vi "ABB locked rotor results.vi"(0 "Rated Current":dbl, 9 "Locked rotor test results":dbl[][](array[numeric])) -> (2 "PFr":dbl, 3 "I AVr":dbl, 4 "IUr":dbl, 6 "IVr":dbl, 8 "PWr":dbl, 10 "IWr":dbl, 13 "V AVr":dbl, 14 "Graph":T1, 15 "Max Value":dbl)   [LabVIEW 2017]
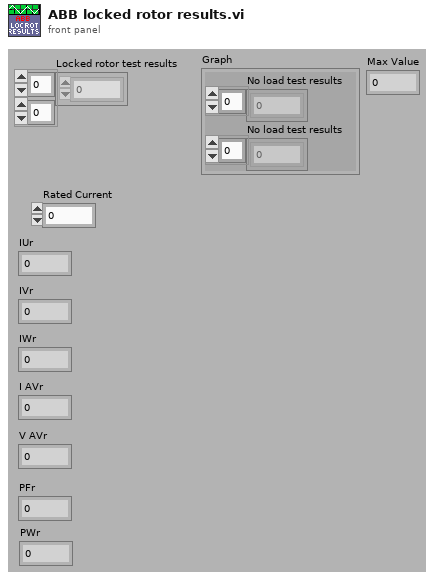
[diagram p1: front panel]
types:
  T1 = cluster{"No load test results":dbl[], "No load test results":dbl[]}
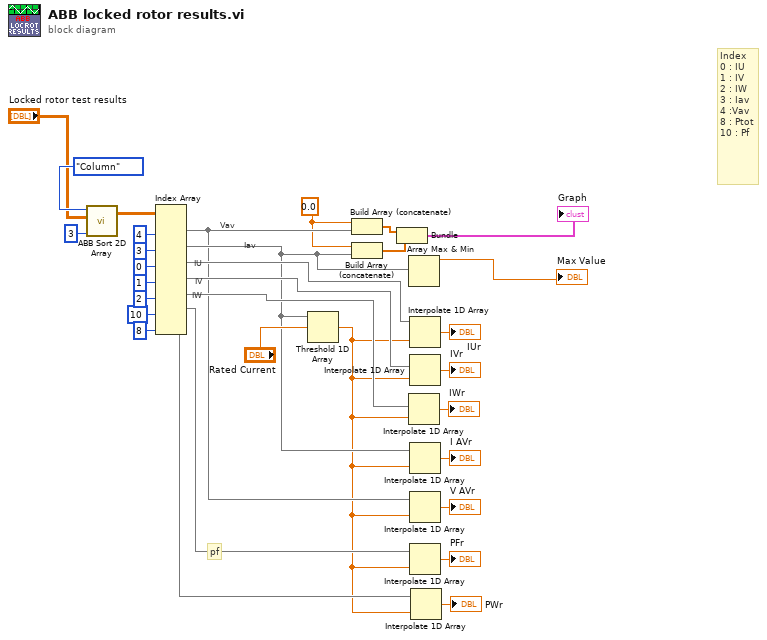
[diagram p0: block diagram]
diagram:
  w1 = 0.0
  # "pf"
  # "IW"
  # "IV"
  # "IU"
  # "Iav"
  # "Vav"
  # "Index\n0 : IU\n1 : IV\n2 : IW\n3 : Iav\n4 :Vav\n8 : Ptot\n10 : Pf"
  n1 = call "ABB Sort 2D Array.vi"("Column/Row to Sort By"=u32 3, "Unsorted 2D Array"="Locked rotor test results", "Sort by"=enum16{"Column", "Row"}."Column") -> ("Sorted 2D Array"=w22:dbl[][])  [unwired: 4 in]
  n2 = Index Array(array=w22, index (col) #1=4 ("disabled index (col)"), index (col) #2=3 ("index (col)"), index (col) #3=0 ("index (col)"), index (col) #4=1 ("index (col)"), index (col) #5=2 ("index (col)"), index (col) #6=10 ("index (col)"), index (col) #7=8 ("index (col)")) -> (element #1=w11:dbl[], element #2=w14:dbl[], element #3=w20:dbl[], element #4=w19:dbl[], element #5=w18:dbl[], element #6=w9:dbl[], element #7=w5:dbl[])  [unwired: 7 in]
  n3 = Threshold 1D Array(2:"Rated Current", 3:w14) -> (0:w4:dbl)  [unwired: 1 in]
  n4 = Build Array (concatenate)(w1, w11) -> (w3:dbl[])
  n5 = Build Array (concatenate)(w1, w14) -> (w2:dbl[])
  n6 = Bundle(w3, w2) -> (→"Graph":cluster{dbl[], dbl[]})  [unwired: 1 in]
  n7 = Array Max & Min(array=w14) -> (max value=→"Max Value":dbl)  [unwired: 3 out]
  n8 = Interpolate 1D Array(1:w4, 2:w18) -> (0:→"IWr":dbl)
  n9 = Interpolate 1D Array(1:w4, 2:w20) -> (0:→"IUr":dbl)
  n10 = Interpolate 1D Array(1:w4, 2:w19) -> (0:→"IVr":dbl)
  n11 = Interpolate 1D Array(1:w4, 2:w14) -> (0:→"I AVr":dbl)
  n12 = Interpolate 1D Array(1:w4, 2:w11) -> (0:→"V AVr":dbl)
  n13 = Interpolate 1D Array(1:w4, 2:w9) -> (0:→"PFr":dbl)
  n14 = Interpolate 1D Array(1:w4, 2:w5) -> (0:→"PWr":dbl)
